vi "Update.vi"(8 "error in (no error)":errorcluster, 11 "Pong in":refnum<class "Pong.lvclass">) -> (0 "error out":errorcluster, 3 "Pong out":refnum<class "Pong.lvclass">)   [LabVIEW 2019, in "RT_Game.lvlib" / "Pong.lvclass"]
uses:
  Pong.lvclass
  C:/Users/FreshBob/Dropbox/VIs/myRIO_GameConsole/RT/RT_Game/Game/Game.lvclass
  Game/Game.lvclass/Game.ctl
  Game/Read State.vi
  Game/Game.lvclass
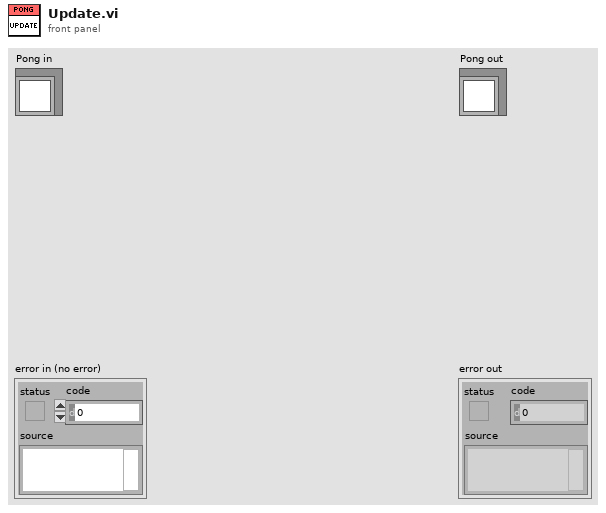
[diagram p1: front panel]
types:
  T1 = typedef "RT_Game.lvlib/Game.lvclass/States.ctl" = enum16{"Init", "Restart", "Menu", "Game", "Resume", "ToggleSingleplayer", "LoadNextGame", "ExitToMenu", "NewHighscore", "GameOver", "SlideOut"}
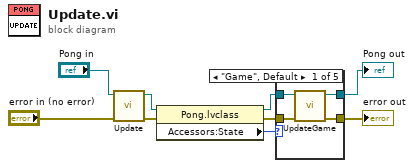
[diagram p0: block diagram]
diagram:
  n1 = call-parent "Update.vi"("error in (no error)"="error in (no error)", "Game in"="Pong in") -> ("error out"=w9:errorcluster, "Game out"=w3:refnum<class "Pong.lvclass">)  [unwired: 8 in]
  n2 = property class="Pong.lvclass"(reference=w3, error in=w9) -> (reference out=w2:refnum<class "Pong.lvclass">, error out=w4:errorcluster, "Accessors:State"=w1:T1)
  n3 = case shown="\"Game\", Default" w1 {
    tunnel: w4 -> [w13 w14 w16 w18 w20]
    tunnel: [w12 w14 w16 w18 w20] -> w6
    tunnel: w2 -> [w11 w15 w17 w19 w21]
    tunnel: [w10 w15 w17 w19 w21] -> w5
    frame "Game", Default {
      n4 = call "UpdateGame.vi"("error in (no error)"=w13, "Pong in"=w11) -> ("error out"=w12:errorcluster, "Pong out"=w10:refnum<class "Pong.lvclass">)  [unwired: 8 in]
    }
    frame "Restart" {
    }
    frame "Menu" {
    }
    frame "SlideOut" {
    }
    frame "Init" {
    }
  }
  "error out" <- w6
  "Pong out" <- w5
